vi "ArmCurlSystem.vi"(8 "Reset Encoder":bool, 9 "Elbow Down":bool, 10 "Elbow Up":bool, 11 "Should Speed":dbl) -> ()   [LabVIEW 2018]
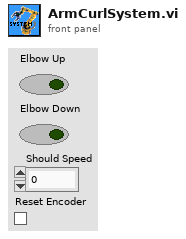
[diagram p1: front panel]
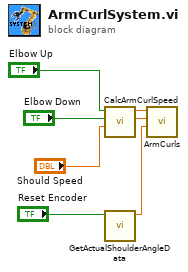
[diagram p0: block diagram]
diagram:
  n1 = call "CalcArmCurlSpeed.vi"("Curl Speed"="Should Speed", "Elbow Down"="Elbow Down", "Elbow Up"="Elbow Up") -> ("Elbow Speed"=w7:dbl, "Shoulder Speed"=w2:dbl)  [unwired: 7 in]
  n2 = call "GetActualShoulderAngleData.vi"("Reset Encoder"="Reset Encoder") -> ("Encoder Angle (deg)"=w1:dbl)  [unwired: 9 in, 1 out]
  n3 = call "ArmCurls.vi"("Actual Shoulder Angle (deg)"=w1, "Elbow Speed"=w7, "shoulder speed (deg/s)"=w2) -> ()  [unwired: 9 in]
